vi "smart decimate .vi"(7 "number of 2D grid points":i32=300, 8 "complex region":T1={"max re"=0.984067684418521, "min re"=-2.0159323155814786, "max im"=3.076570113964653, "min im"=0.06786753047429528, "delta re"=2.9999999999999996, "delta im"=3.008702583490358, "center re"=-0.5159323155814788, "delta  z"=1.5722188222194742+0.0i, "center im"=0.0, "center z"=0.0+0.0i, "d im"=0.0, "d re"=0.0, "d z"=0.0+0.0i}, 9 "omega in":dbl[](array[numeric]), 10 "decimation threshold":i32=3, 11 "z in":cdb[](array[numeric])) -> (1 "decimated omega":dbl[](array[numeric]), 3 "decimated z":cdb[](array[numeric]))   [LabVIEW 2021]
uses:
  complex region.ctl
panel:
  in  "x + iy":cdb[](array[numeric])
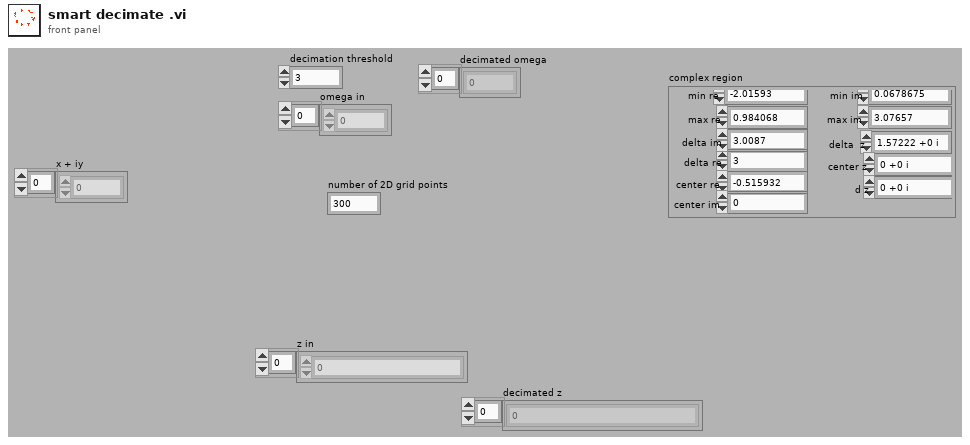
[diagram p1: front panel]
types:
  T1 = typedef "complex region.ctl" = cluster{"max re":dbl, "min re":dbl, "max im":dbl, "min im":dbl, "delta re":dbl, "delta im":dbl, "center re":dbl, "delta  z":cdb, "center im":dbl, "center z":cdb, "d im":dbl, "d re":dbl, "d z":cdb}
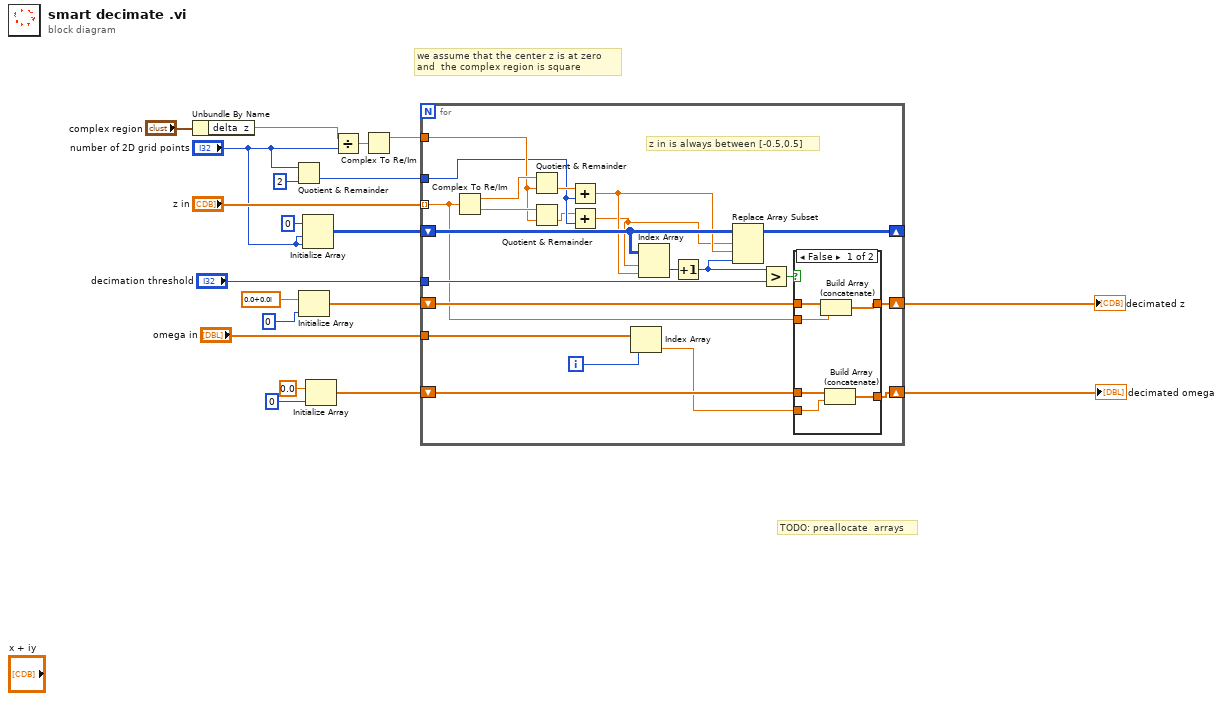
[diagram p0: block diagram]
diagram:
  # "TODO: preallocate  arrays"
  # "we assume that the center z is at zero \nand  the complex region is square"
  n1 = Unbundle By Name("complex region") -> ("delta  z"=w5:cdb)
  n2 = Quotient & Remainder(x="number of 2D grid points", y=2) -> (floor(x/y)=w1:i32)  [unwired: 1 out]
  n3 = Initialize Array(cdb 0.0+0.0i ("element"), 0 ("element")) -> (w17:cdb[])
  n4 = Initialize Array(i16 0 ("element"), "number of 2D grid points", "number of 2D grid points") -> (w16:i16[][])
  n5 = Initialize Array(0.0 ("element"), 0 ("element")) -> (w9:dbl[])
  n6 = Divide(x=w5, y="number of 2D grid points") -> (x/y=w6:cdb)
  n7 = Complex To Re/Im(x + iy=w6) -> (x=w4:dbl)  [unwired: 1 out]
  n8 = for {
    shift-right: [w37] -> w15
    shift-left: w17 -> [w36]
    tunnel: "z in" -> [w26] mode=indexing
    shift-right: [w40] -> _
    shift-left: w16 -> [w41]
    tunnel: "decimation threshold" -> [w35]
    tunnel: "omega in" -> [w34]
    shift-right: [w31] -> w8
    shift-left: w9 -> [w32]
    tunnel: w4 -> [w27]
    tunnel: w1 -> [w22]
    i -> [w33]
    # "z in is always between [-0.5,0.5]"
    n9 = Complex To Re/Im(x + iy=w26) -> (x=w29:dbl, y=w28:dbl)
    n10 = Quotient & Remainder(x=w29, y=w27) -> (floor(x/y)=w24:dbl)  [unwired: 1 out]
    n11 = Quotient & Remainder(x=w28, y=w27) -> (floor(x/y)=w21:dbl)  [unwired: 1 out]
    n12 = Add(x=w24, y=w22) -> (x+y=w25:dbl)
    n13 = Add(x=w21, y=w22) -> (x+y=w23:dbl)
    n14 = Index Array(array=w34, index=w33) -> (element=w30:dbl)
    n15 = Index Array(array=w41, index (row)=w23, index (col)=w25) -> (element=w42:i16)
    n16 = Increment(x=w42) -> (x+1=w39:i16)
    n17 = Replace Array Subset(array=w41, new element=w39, index (row)=w23, index (col)=w25) -> (w40:i16[][])
    n18 = Greater?(x=w39, y=w35) -> (0:w38:bool)
    n19 = case shown="False" w38 {
      tunnel: [w46 w50] -> w37
      tunnel: w36 -> [w48 w50]
      tunnel: w26 -> [w47 _]
      tunnel: w32 -> [w45 w49]
      tunnel: [w44 w49] -> w31
      tunnel: w30 -> [w43 _]
      frame False {
        n20 = Build Array (concatenate)(w48, w47) -> (w46:cdb[])
        n21 = Build Array (concatenate)(w45, w43) -> (w44:dbl[])
      }
      frame True {
      }
    }
  }
  "decimated z" <- w15
  "decimated omega" <- w8
